vi "Trigger Response.vi"(7 "History length":i32=20, 8 "Triggers":T1=enum."End Trial", 11 "State Output":T2) -> (3 "Output":variant)   [LabVIEW 2010]
uses:
  Matlab API/Matlab API.lvlib
  Matlab API/Matlab Param Array to DBL.vi
  Matlab API/Matlab Param Array to I32.vi
  Trial Based Experiment.lvsc/Outputs.ctl
  Trial Based Experiment.lvsc
  TYPE - State triggers.ctl
  TrialBasedExperimentObject/TrialBasedExperiment.lvclass
panel:
  out "fixationRadius":dbl
  out "joystickThreshold":dbl
  out "trial type":i32
  in  "Number conditions":i32=2
  out "Right":dbl(graph)
  out "Left":dbl(graph)
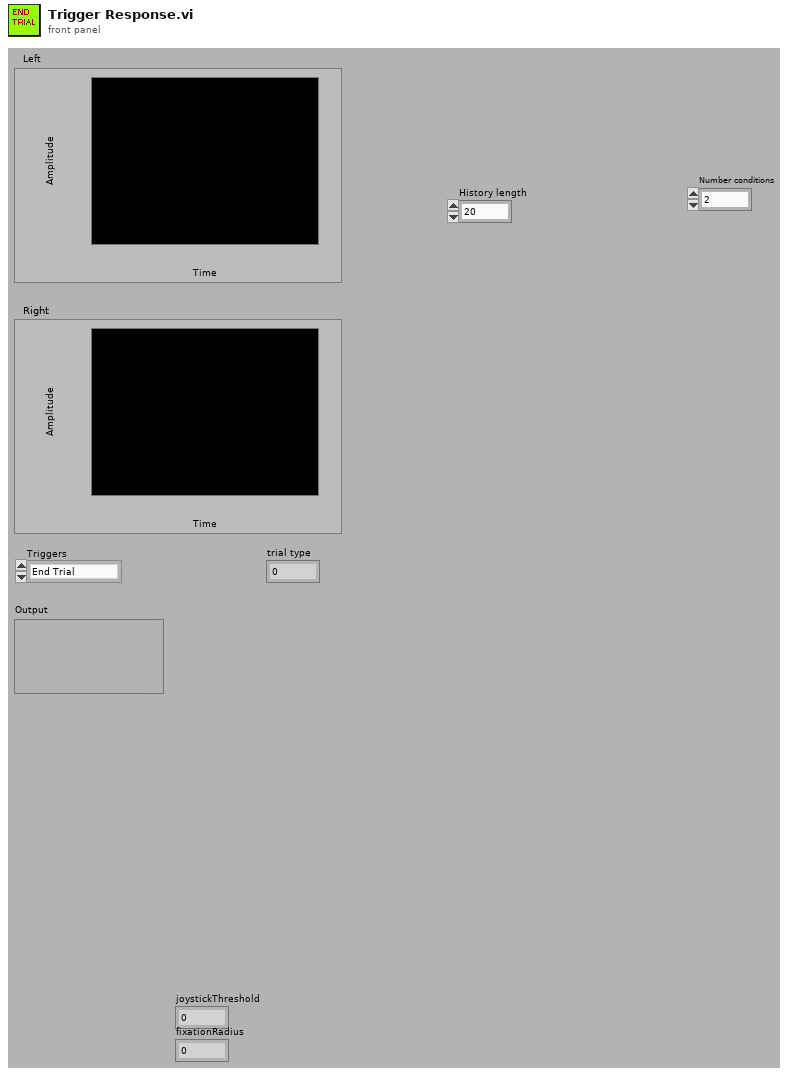
[diagram p1: front panel]
types:
  T1 = typedef "TYPE - State triggers.ctl" = enum16{"Start Session", "Start Trial", "Intertrial", "Acquire Fixation", "Delay Period", "Response Period", "Reward", "Abort Trial", "End Trial"}
  T2 = typedef "Trial Based Experiment.lvsc/Outputs.ctl" = cluster{"Experiment":refnum<class "TrialBasedExperiment.lvclass">, "Timeout":dbl, "error out":errorcluster}
  T3 = cluster{"Trial Type":i32, "Joystick Threshold":dbl, "Fixation Radius":dbl}
  T4 = typedef "TYPE - Trial Outcome.ctl" = enum16{"Aborted", "Correct", "Incorrect"}
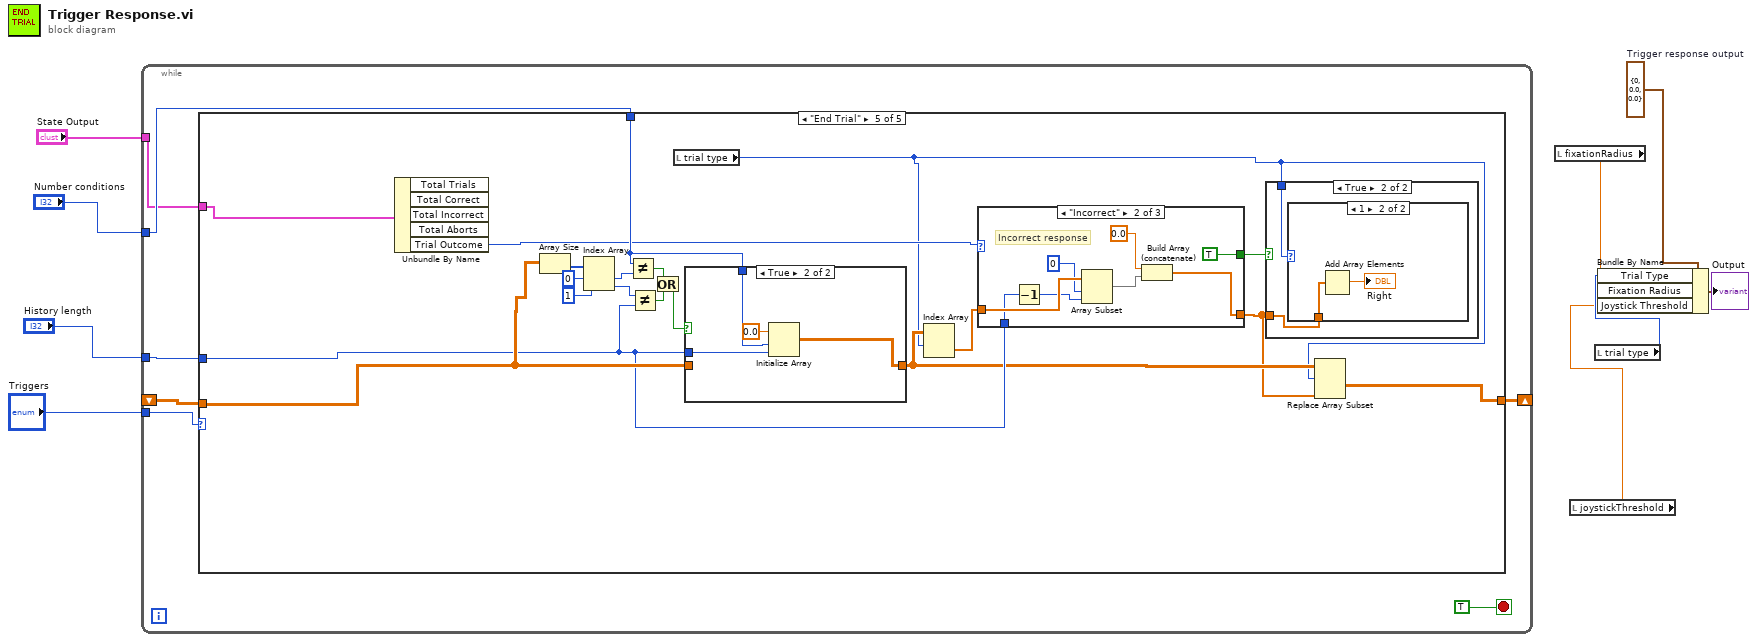
[diagram p0: block diagram]
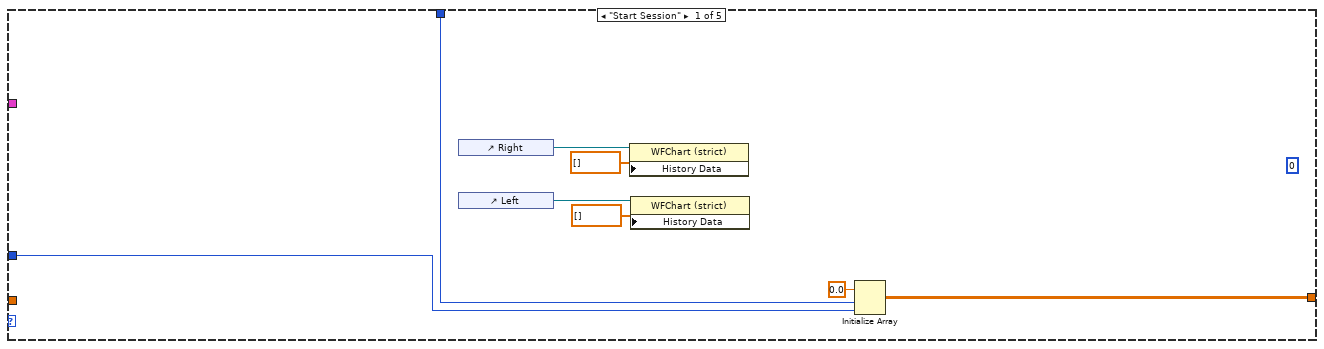
[diagram p2: hidden frame]
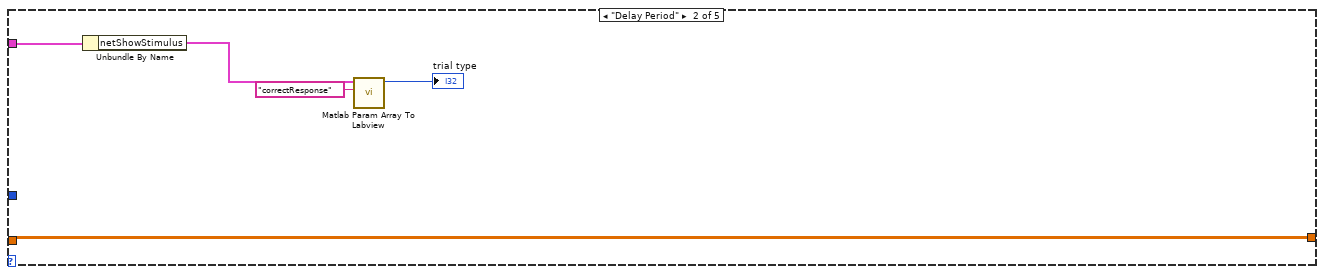
[diagram p3: hidden frame]
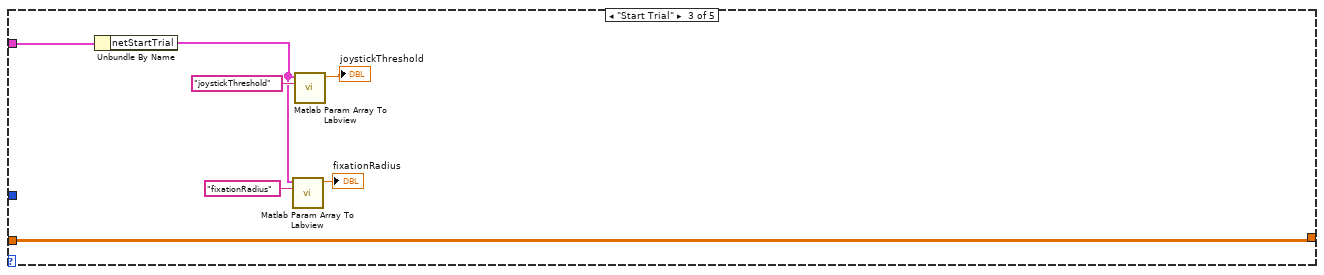
[diagram p4: hidden frame]
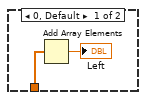
[diagram p7: hidden frame]
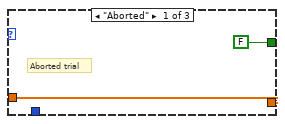
[diagram p9: hidden frame]
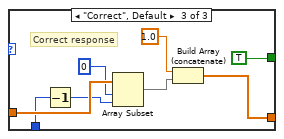
[diagram p10: hidden frame]
diagram:
  w1 = T3 {"Trial Type"=0, "Joystick Threshold"=0.0, "Fixation Radius"=0.0}  # Trigger response output
  n1 = while {
    shift-right: [w15] -> _
    shift-left: _ -> [w14]
    tunnel: "History length" -> [w13]
    tunnel: "Number conditions" -> [w12]
    tunnel: "Triggers" -> [w11]
    tunnel: "State Output" -> [w10]
    stop <- TRUE stop-if-true
    n2 = case shown="\"End Trial\"" w11 {
      tunnel: [w21 w29 w30 w37 w56] -> w15
      tunnel: w14 -> [_ w29 w30 w37 w55]
      tunnel: w13 -> [w19 _ _ _ w54]
      tunnel: w12 -> [w20 _ _ _ w53]
      tunnel: w10 -> [_ w28 w36 _ w52]
      frame "Start Session" {
        (unwired) 0 ("data")
        n3 = control-ref of="Right"() -> (w17:refnum<vi>)
        n4 = control-ref of="Left"() -> (w18:refnum<vi>)
        n5 = property on="Property Node" class="WFChart (strict)"(reference=w17, "History Data"=dbl[] []) -> ()  [unwired: 1 in, 2 out]
        n6 = property on="Property Node" class="WFChart (strict)"(reference=w18, "History Data"=dbl[] []) -> ()  [unwired: 1 in, 2 out]
        n7 = Initialize Array(0.0 ("element"), w20, w19) -> (w21:dbl[][])
      }
      frame "Delay Period" {
        n8 = Unbundle By Name(w28) -> ("netShowStimulus"=w27:cluster{"Name":string, "Data":variant}[])
        n9 = call-poly "Matlab Param Array To Labview.vi"("Name"="correctResponse", "Matlab Param Array"=w27) -> ("data"=→"trial type":i32)  [unwired: 8 in, 1 out]
      }
      frame "Start Trial" {
        n10 = Unbundle By Name(w36) -> ("netStartTrial"=w33:cluster{"Name":string, "Data":variant}[])
        n11 = call-poly "Matlab Param Array To Labview.vi"("Name"="fixationRadius", "Matlab Param Array"=w33) -> ("data"=→"fixationRadius":dbl)  [unwired: 8 in, 1 out]
        n12 = call-poly "Matlab Param Array To Labview.vi"("Name"="joystickThreshold", "Matlab Param Array"=w33) -> ("data"=→"joystickThreshold":dbl)  [unwired: 8 in, 1 out]
      }
      frame "Response Period", Default {
      }
      frame "End Trial" {
        n13 = Unbundle By Name(w52) -> ("Trial Outcome"=w51:T4)  [unwired: 4 out]
        n14 = Array Size(array=w55) -> (size(s)=w49:i32[])
        n15 = Index Array(array=w49, index #1=0 ("index"), index #2=1 ("index")) -> (element #1=w45:i32, element #2=w44:i32)
        n16 = Not Equal?(x=w53, y=w45) -> (x != y?=w43:bool)
        n17 = Not Equal?(x=w44, y=w54) -> (x != y?=w42:bool)
        n18 = Or(x=w43, y=w42) -> (x .or. y?=w41:bool)
        n19 = local read "trial type"() -> (w38:i32)
        n20 = case shown="True" w41 {
          tunnel: w55 -> [w63 _]
          tunnel: [w63 w64] -> w47
          tunnel: w54 -> [_ w66]
          tunnel: w53 -> [_ w65]
          frame False {
          }
          frame True {
            n21 = Initialize Array(0.0 ("element"), w65, w66) -> (w64:dbl[][])
          }
        }
        n22 = Index Array(array=w47, index (row)=w38) -> (element=w50:dbl[])  [unwired: 1 in]
        n23 = case shown="\"Incorrect\"" w51 {
          tunnel: w50 -> [w69 w77 w85]
          tunnel: [w69 w71 w79] -> w40
          tunnel: w54 -> [_ w75 w83]
          tunnel: [FALSE TRUE TRUE] -> w39
          frame "Aborted" {
            # "Aborted trial"
          }
          frame "Incorrect" {
            # "Incorrect response"
            n24 = Decrement(x=w75) -> (x-1=w74:i32)
            n25 = Array Subset(array=w77, index=0, length=w74) -> (w73:dbl[])
            n26 = Build Array (concatenate)(0.0 ("element"), w73) -> (w71:dbl[])
          }
          frame "Correct", Default {
            # "Correct response"
            n27 = Decrement(x=w83) -> (x-1=w82:i32)
            n28 = Array Subset(array=w85, index=0, length=w82) -> (w81:dbl[])
            n29 = Build Array (concatenate)(1.0 ("element"), w81) -> (w79:dbl[])
          }
        }
        n30 = case shown="True" w39 {
          tunnel: w40 -> [_ w58]
          tunnel: w38 -> [_ w57]
          frame False {
          }
          frame True {
            n31 = case shown="1" w57 {
              tunnel: w58 -> [w59 w61]
              frame 0, Default {
                n32 = Add Array Elements(numeric array=w59) -> (sum=→"Left":dbl)
              }
              frame 1 {
                n33 = Add Array Elements(numeric array=w61) -> (sum=→"Right":dbl)
              }
            }
          }
        }
        n34 = Replace Array Subset(array=w47, new element=w40, index (row)=w38) -> (w56:dbl[][])  [unwired: 1 in]
      }
    }
  }
  n35 = local read "fixationRadius"() -> (w4:dbl)
  n36 = local read "joystickThreshold"() -> (w2:dbl)
  n37 = local read "trial type"() -> (w3:i32)
  n38 = Bundle By Name(cluster=w1, "Trial Type"=w3, "Fixation Radius"=w4, "Joystick Threshold"=w2) -> (→"Output":T3)
